vi "Untitled 7 (SubVI).vi"(8 "error in (no error)":errorcluster, 10 "Tag name":string, 11 "body":string) -> (0 "error out":errorcluster, 3 "MonitorInstanceResponse":T1)   [LabVIEW 2012, in "AWS_EC2.lvlib" / "AWS_EC2.lvclass"]
uses:
  AWS_EC2.lvclass
  Response Typedefs/MonitorInstancesResult.ctl
  AWS Core Lib/VI Source/XML Parser/AWS_XML Parser.lvlib
  AWS_EC2.lvlib
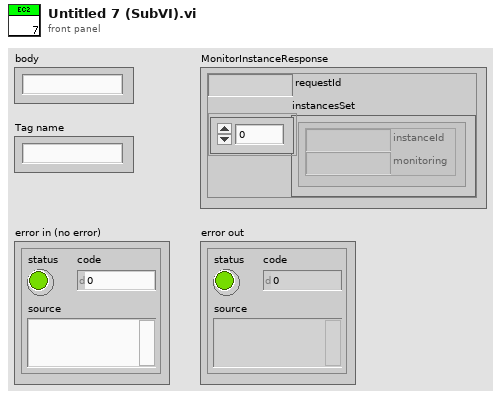
[diagram p1: front panel]
types:
  T1 = typedef "AWS_EC2.lvlib/MonitorInstancesResult.ctl" = cluster{"requestId":string, "instancesSet":cluster{"instanceId":string, "monitoring":string}[]}
  T2 = cluster{"instanceId":string, "monitoring":string}[]
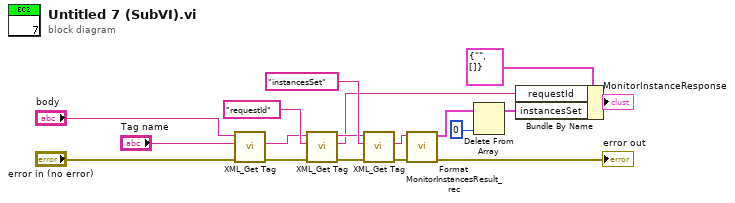
[diagram p0: block diagram]
diagram:
  n1 = call "XML_Get Tag.vi"("error in (no error)"="error in (no error)", "Tag name"="Tag name", "XML String in"="body") -> ("error out"=w8:errorcluster, "Tag value"=w5:string)  [unwired: 4 in, 3 out]
  n2 = call "XML_Get Tag.vi"("error in (no error)"=w8, "Tag name"="requestId", "XML String in"=w5) -> ("error out"=w9:errorcluster, "Tag value"=w7:string, "XML String dup"=w10:string)  [unwired: 4 in, 2 out]
  n3 = call "XML_Get Tag.vi"("error in (no error)"=w9, "Tag name"="instancesSet", "XML String in"=w10) -> ("error out"=w13:errorcluster, "Tag value"=w12:string)  [unwired: 4 in, 3 out]
  n4 = call "Format MonitorInstancesResult_rec.vi"("error in (no error)"=w13, "XML String"=w12) -> ("Error Out"=→"error out":errorcluster, "Array"=w17:T2)  [unwired: 8 in]
  n5 = Delete From Array(array=w17, index=0) -> (array with subset deleted=w18:T2)  [unwired: 1 in, 1 out]
  n6 = Bundle By Name(cluster=T1 {"requestId"="", "instancesSet"=[]} ("MonitorInstanceResponse"), "requestId"=w7, "instancesSet"=w18) -> (→"MonitorInstanceResponse":T1)
